vi "RevertMapX.vi"(11 "Tilenumbers":u32[][](array[numeric])) -> (3 "Array":u32[][](array[numeric]))   [LabVIEW 2019, in "RT_Game.lvlib" / "Engine.lvclass"]
uses:
  Engine.lvclass
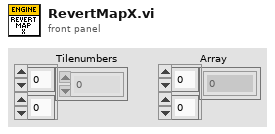
[diagram p1: front panel]
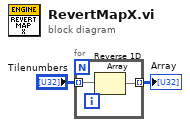
[diagram p0: block diagram]
diagram:
  n1 = for {
    tunnel: "Tilenumbers" -> [w4] mode=indexing
    tunnel: [w3] -> w2 mode=indexing
    n2 = Reverse 1D Array(array=w4) -> (reversed array=w3:u32[])
  }
  "Array" <- w2
